vi "Query.vi"(7 "Return":bool, 8 "error in (no error)":errorcluster, 10 "Command":string, 11 "E5071C in":refnum<class "E5071C.lvclass">) -> (0 "error out":errorcluster, 2 "read buffer":string, 3 "E5071C out":refnum<class "E5071C.lvclass">)   [LabVIEW 2020, in "E5071C.lvlib" / "E5071C.lvclass"]
uses:
  E5071C.lvclass
  E5071C.lvclass/E5071C.ctl
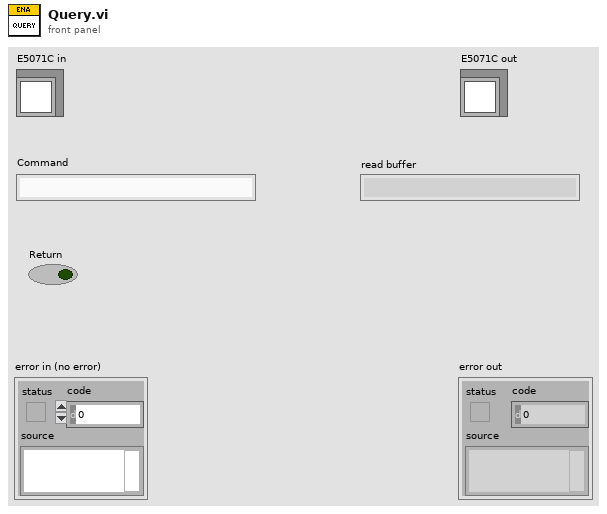
[diagram p1: front panel]
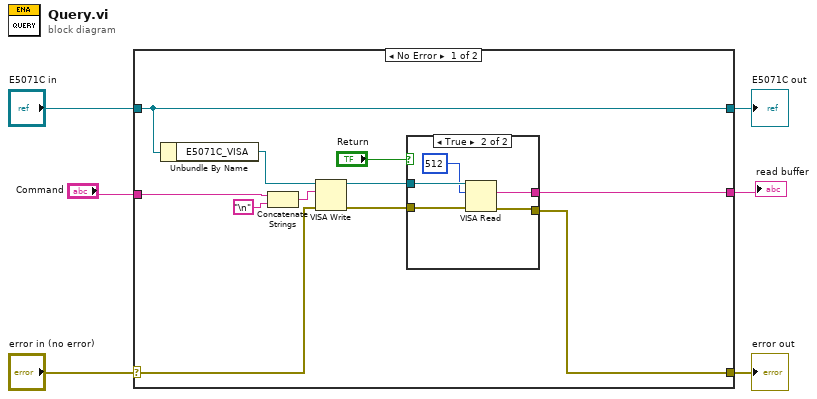
[diagram p0: block diagram]
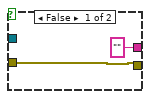
[diagram p2: hidden frame]
diagram:
  n1 = case shown="No Error" "error in (no error)" {
    selector: "error in (no error)" -> [w8 w26]
    tunnel: [w7 w26] -> w5
    tunnel: [w17 w25] -> w3
    tunnel: "E5071C in" -> [w17 w25]
    tunnel: "Command" -> [w14 _]
    tunnel: [w9 _] -> w1
    frame No Error {
      n2 = Unbundle By Name(w17) -> ("E5071C_VISA"=w16:refnum<visa-resource-name>)
      n3 = Concatenate Strings(w14, "\n") -> (w13:string)
      n4 = VISA Write(VISA resource name=w16, write buffer=w13, error in (no error)=w8) -> (VISA resource name out=w11:refnum<visa-resource-name>, error out=w12:errorcluster)  [unwired: 1 out]
      n5 = case shown="True" "Return" {
        tunnel: w12 -> [w18 w24]
        tunnel: w11 -> [_ w23]
        tunnel: ["" ("read buffer") w21] -> w9
        tunnel: [w18 w20] -> w7
        frame False {
        }
        frame True {
          n6 = VISA Read(VISA resource name=w23, byte count=u32 512, error in (no error)=w24) -> (read buffer=w21:string, error out=w20:errorcluster)  [unwired: 2 out]
        }
      }
    }
    frame Error {
    }
  }
  "error out" <- w5
  "E5071C out" <- w3
  "read buffer" <- w1
